vi "MIPI_RFEE_Create Patterns and save to HWS file.vi"(1 "SetID Pin State":u8(ring) items=["0", "1", "Z"], 2 "Mode":enum16{"Write", "Read"}(ring), 5 "file path":path=path "C:/Users/user/Documents/AD2240/Waveforms/RFFE6", 12 "Save .HWS?":bool, 13 "Filename":string) -> ()   [LabVIEW 2013]
doc: "This VI demonstaits how to write to and read back data from a MIPI device. To run this VI:\n1) Change Resource name to the name of your HSDIO card\n2) The MIPI clock will run at <Sample Clock Rate>/<Oversample Factor>. This is 26 MHz (full rate). If your device should be run at a slower rate, decrease the sample clock rate and (or) increase the oversample rate.\n3. At 104MHz, the RTD value should be ~5 for a 1.5 meter cable. If you are running at a different clock rate or using a different length cable, adjust the RTD Compensation value so the MIPI data is stable at the falling edge of the clock. If you need futher timing adjustment, consider setting the data position to \"Delay from Sample Clock Rising Edge\" and configuring this delay."
uses:
  MIPI_RFFE/Ctrls/Configuration.ctl
  MIPI_RFFE/Ctrls/ClockDataChannels.ctl
  MIPI_RFFE/Ctrls/RegReadWrite.ctl
  MIPI_RFFE/Ctrls/ExtendedRegReadWrite.ctl
  <vilib>/Waveform/DWDTOps.llb/Digital Pattern Generator (Single Value).vi
  <vilib>/Waveform/DWDTOps.llb/DWDT Append Digital Signals.vi
  <vilib>/Waveform/DWDTOps.llb/DWDT Append Digital Samples.vi
panel:
  in  "Write Data":T1 {"Register" format="%.0x"; "Slave Address" max=15 format="%.0x"}
  out "Digital Waveform Graph":digitalwaveform(graph)={"t0"=timestamp(3585852840.1106524 s since 1904-01-01), "dt"=5e-07, "Y"={"transitions"=[], "data"=[[1, 0, 1, 0], [1, 0, 1, 0], [1, 0, 1, 0], [1, 0, 1, 0], [1, 0, 1, 0], [1, 0, 1, 0], [1, 0, 1, 0], [1, 0, 1, 0], [0, 0, 0, 0], [0, 0, 0, 0], [0, 0, 0, 0], [0, 0, 0, 0], [0, 0, 0, 0], [0, 0, 0, 0], [0, 0, 0, 0], [0, 0, 0, 0], [0, 1, 0, 1], [0, 1, 0, 1], [0, 1, 0, 1], [0, 1, 0, 1], [0, 0, 0, 0], [0, 0, 0, 0], [0, 0, 0, 0], [0, 0, 0, 0], [1, 1, 1, 1], [1, 1, 1, 1], [1, 1, 1, 1], [1, 1, 1, 1], [1, 0, 1, 0], [1, 0, 1, 0], [1, 0, 1, 0], [1, 0, 1, 0], [1, 1, 1, 1], [1, 1, 1, 1], [1, 1, 1, 1], [1, 1, 1, 1], [1, 0, 1, 0], [1, 0, 1, 0], [1, 0, 1, 0], [1, 0, 1, 0], [0, 1, 0, 1], [0, 1, 0, 1], [0, 1, 0, 1], [0, 1, 0, 1], [0, 0, 0, 0], [0, 0, 0, 0], [0, 0, 0, 0], [0, 0, 0, 0], [0, 1, 0, 1], [0, 1, 0, 1], [0, 1, 0, 1], [0, 1, 0, 1], [0, 0, 0, 0], [0, 0, 0, 0], [0, 0, 0, 0], [0, 0, 0, 0], [1, 1, 1, 1], [1, 1, 1, 1], [1, 1, 1, 1], [1, 1, 1, 1], [1, 0, 1, 0], [1, 0, 1, 0], [1, 0, 1, 0], [1, 0, 1, 0], [0, 1, 0, 1], [0, 1, 0, 1], [0, 1, 0, 1], [0, 1, 0, 1], [0, 0, 0, 0], [0, 0, 0, 0], [0, 0, 0, 0], [0, 0, 0, 0], [1, 1, 1, 1], [1, 1, 1, 1], [1, 1, 1, 1], [1, 1, 1, 1], [1, 0, 1, 0], [1, 0, 1, 0], [1, 0, 1, 0], [1, 0, 1, 0], [1, 1, 1, 1], [1, 1, 1, 1], [1, 1, 1, 1], [1, 1, 1, 1], [1, 0, 1, 0], [1, 0, 1, 0], [1, 0, 1, 0], [1, 0, 1, 0], [1, 1, 1, 1], [1, 1, 1, 1], [1, 1, 1, 1], [1, 1, 1, 1], [1, 0, 1, 0], [1, 0, 1, 0], [1, 0, 1, 0], [1, 0, 1, 0], [0, 1, 0, 1], [0, 1, 0, 1], [0, 1, 0, 1], [0, 1, 0, 1], [0, 0, 0, 0], [0, 0, 0, 0], [0, 0, 0, 0], [0, 0, 0, 0], [0, 1, 0, 1], [0, 1, 0, 1], [0, 1, 0, 1], [0, 1, 0, 1], [0, 0, 0, 0], [0, 0, 0, 0], [0, 0, 0, 0], [0, 0, 0, 0], [1, 1, 1, 1], [1, 1, 1, 1], [1, 1, 1, 1], [1, 1, 1, 1], [1, 0, 1, 0], [1, 0, 1, 0], [1, 0, 1, 0], [1, 0, 1, 0], [1, 1, 1, 1], [1, 1, 1, 1], [1, 1, 1, 1], [1, 1, 1, 1], [1, 0, 1, 0], [1, 0, 1, 0], [1, 0, 1, 0], [1, 0, 1, 0], [0, 1, 0, 1], [0, 1, 0, 1], [0, 1, 0, 1], [0, 1, 0, 1], [0, 0, 0, 0], [0, 0, 0, 0], [0, 0, 0, 0], [0, 0, 0, 0], [0, 1, 0, 1], [0, 1, 0, 1], [0, 1, 0, 1], [0, 1, 0, 1], [0, 0, 0, 0], [0, 0, 0, 0], [0, 0, 0, 0], [0, 0, 0, 0], [0, 1, 0, 1], [0, 1, 0, 1], [0, 1, 0, 1], [0, 1, 0, 1], [0, 0, 0, 0], [0, 0, 0, 0], [0, 0, 0, 0], [0, 0, 0, 0], [0, 1, 0, 1], [0, 1, 0, 1], [0, 1, 0, 1], [0, 1, 0, 1], [0, 0, 0, 0], [0, 0, 0, 0], [0, 0, 0, 0], [0, 0, 0, 0], [0, 1, 0, 1], [0, 1, 0, 1], [0, 1, 0, 1], [0, 1, 0, 1], [0, 0, 0, 0], [0, 0, 0, 0], [0, 0, 0, 0], [0, 0, 0, 0], [0, 1, 0, 1], [0, 1, 0, 1], [0, 1, 0, 1], [0, 1, 0, 1], [0, 0, 0, 0], [0, 0, 0, 0], [0, 0, 0, 0], [0, 0, 0, 0], [0, 1, 0, 1], [0, 1, 0, 1], [0, 1, 0, 1], [0, 1, 0, 1], [0, 0, 0, 0], [0, 0, 0, 0], [0, 0, 0, 0], [0, 0, 0, 0], [0, 1, 0, 1], [0, 1, 0, 1], [0, 1, 0, 1], [0, 1, 0, 1], [0, 0, 0, 0], [0, 0, 0, 0], [0, 0, 0, 0], [0, 0, 0, 0], [0, 1, 0, 1], [0, 1, 0, 1], [0, 1, 0, 1], [0, 1, 0, 1], [0, 0, 0, 0], [0, 0, 0, 0], [0, 0, 0, 0], [0, 0, 0, 0], [1, 0, 1, 0], [1, 0, 1, 0], [1, 0, 1, 0], [1, 0, 1, 0], [1, 0, 1, 0], [1, 0, 1, 0], [1, 0, 1, 0], [1, 0, 1, 0], [0, 0, 0, 0], [0, 0, 0, 0], [0, 0, 0, 0], [0, 0, 0, 0], [0, 0, 0, 0], [0, 0, 0, 0], [0, 0, 0, 0], [0, 0, 0, 0], [0, 1, 0, 1], [0, 1, 0, 1], [0, 1, 0, 1], [0, 1, 0, 1], [0, 0, 0, 0], [0, 0, 0, 0], [0, 0, 0, 0], [0, 0, 0, 0], [1, 1, 1, 1], [1, 1, 1, 1], [1, 1, 1, 1], [1, 1, 1, 1], [1, 0, 1, 0], [1, 0, 1, 0], [1, 0, 1, 0], [1, 0, 1, 0], [1, 1, 1, 1], [1, 1, 1, 1], [1, 1, 1, 1], [1, 1, 1, 1], [1, 0, 1, 0], [1, 0, 1, 0], [1, 0, 1, 0], [1, 0, 1, 0], [0, 1, 0, 1], [0, 1, 0, 1], [0, 1, 0, 1], [0, 1, 0, 1], [0, 0, 0, 0], [0, 0, 0, 0], [0, 0, 0, 0], [0, 0, 0, 0], [0, 1, 0, 1], [0, 1, 0, 1], [0, 1, 0, 1], [0, 1, 0, 1], [0, 0, 0, 0], [0, 0, 0, 0], [0, 0, 0, 0], [0, 0, 0, 0], [1, 1, 1, 1], [1, 1, 1, 1], [1, 1, 1, 1], [1, 1, 1, 1], [1, 0, 1, 0], [1, 0, 1, 0], [1, 0, 1, 0], [1, 0, 1, 0], [1, 1, 1, 1], [1, 1, 1, 1], [1, 1, 1, 1], [1, 1, 1, 1], [1, 0, 1, 0], [1, 0, 1, 0], [1, 0, 1, 0], [1, 0, 1, 0], [1, 1, 1, 1], [1, 1, 1, 1], [1, 1, 1, 1], [1, 1, 1, 1], [1, 0, 1, 0], [1, 0, 1, 0], [1, 0, 1, 0], [1, 0, 1, 0], [1, 1, 1, 1], [1, 1, 1, 1], [1, 1, 1, 1], [1, 1, 1, 1], [1, 0, 1, 0], [1, 0, 1, 0], [1, 0, 1, 0], [1, 0, 1, 0], [1, 1, 1, 1], [1, 1, 1, 1], [1, 1, 1, 1], [1, 1, 1, 1], [1, 0, 1, 0], [1, 0, 1, 0], [1, 0, 1, 0], [1, 0, 1, 0], [0, 1, 0, 1], [0, 1, 0, 1], [0, 1, 0, 1], [0, 1, 0, 1], [0, 0, 0, 0], [0, 0, 0, 0], [0, 0, 0, 0], [0, 0, 0, 0], [0, 1, 0, 1], [0, 1, 0, 1], [0, 1, 0, 1], [0, 1, 0, 1], [0, 0, 0, 0], [0, 0, 0, 0], [0, 0, 0, 0], [0, 0, 0, 0], [0, 1, 0, 1], [0, 1, 0, 1], [0, 1, 0, 1], [0, 1, 0, 1], [0, 0, 0, 0], [0, 0, 0, 0], [0, 0, 0, 0], [0, 0, 0, 0], [0, 1, 0, 1], [0, 1, 0, 1], [0, 1, 0, 1], [0, 1, 0, 1], [0, 0, 0, 0], [0, 0, 0, 0], [0, 0, 0, 0], [0, 0, 0, 0], [1, 1, 5, 1], [1, 1, 5, 1], [1, 1, 5, 1], [1, 1, 5, 1], [1, 0, 4, 0], [1, 0, 5, 0], [1, 0, 5, 0], [1, 0, 5, 0], [0, 1, 5, 1], [0, 1, 5, 1], [0, 1, 5, 1], [0, 1, 5, 1], [0, 0, 3, 0], [0, 0, 5, 0], [0, 0, 5, 0], [0, 0, 5, 0], [0, 1, 5, 1], [0, 1, 5, 1], [0, 1, 5, 1], [0, 1, 5, 1], [0, 0, 3, 0], [0, 0, 5, 0], [0, 0, 5, 0], [0, 0, 5, 0], [0, 1, 5, 1], [0, 1, 5, 1], [0, 1, 5, 1], [0, 1, 5, 1], [0, 0, 3, 0], [0, 0, 5, 0], [0, 0, 5, 0], [0, 0, 5, 0], [0, 1, 5, 1], [0, 1, 5, 1], [0, 1, 5, 1], [0, 1, 5, 1], [0, 0, 3, 0], [0, 0, 5, 0], [0, 0, 5, 0], [0, 0, 5, 0], [0, 1, 5, 1], [0, 1, 5, 1], [0, 1, 5, 1], [0, 1, 5, 1], [0, 0, 3, 0], [0, 0, 5, 0], [0, 0, 5, 0], [0, 0, 5, 0], [0, 1, 5, 1], [0, 1, 5, 1], [0, 1, 5, 1], [0, 1, 5, 1], [0, 0, 3, 0], [0, 0, 5, 0], [0, 0, 5, 0], [0, 0, 5, 0], [0, 1, 5, 1], [0, 1, 5, 1], [0, 1, 5, 1], [0, 1, 5, 1], [0, 0, 3, 0], [0, 0, 5, 0], [0, 0, 5, 0], [0, 0, 5, 0], [0, 1, 5, 1], [0, 1, 5, 1], [0, 1, 5, 1], [0, 1, 5, 1], [0, 0, 3, 0], [0, 0, 5, 0], [0, 0, 5, 0], [0, 0, 5, 0], [0, 1, 0, 1], [0, 1, 0, 1], [0, 1, 0, 1], [0, 1, 0, 1], [0, 0, 0, 0], [0, 0, 0, 0], [0, 0, 0, 0], [0, 0, 0, 0]]}}
  in  "Configuratation":T2={"Samples to Allocate"=10000, "Oversample Factor"=1, "Clock Channel"=enum."0", "Data Channel"=enum."1"} {"Oversample Factor" min=1 max=254; "Samples to Allocate" min=1}
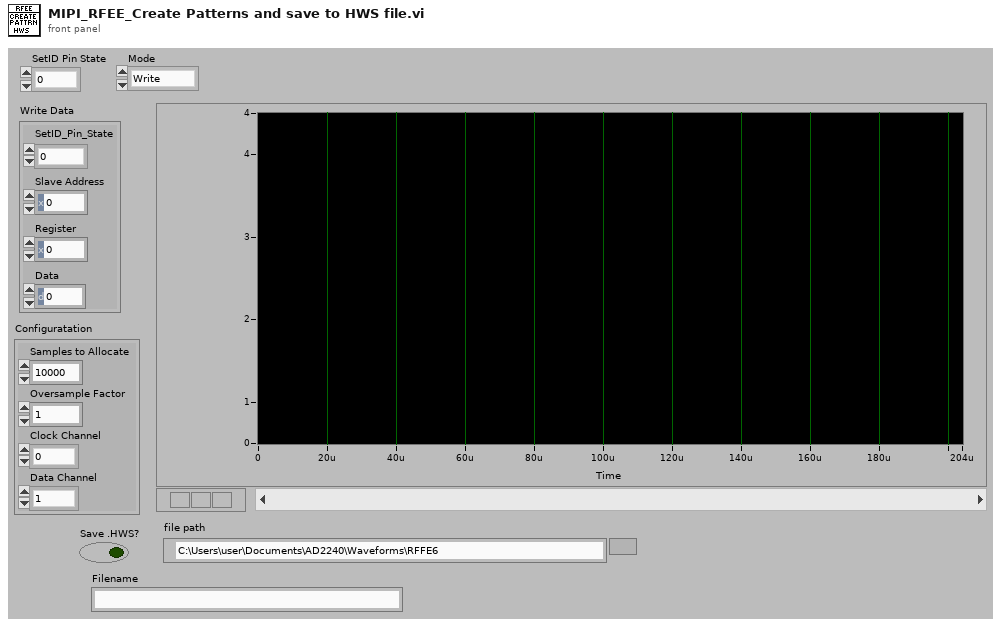
[diagram p1: front panel]
types:
  T1 = typedef "RegReadWrite.ctl" = cluster{"Slave Address":u8, "Register":u8, "Data":u8, "SetID_Pin_State":enum16{"0", "1", "Z"}}
  T2 = typedef "Configuration.ctl" = cluster{"Samples to Allocate":i32, "Oversample Factor":u8, "Clock Channel":T3, "Data Channel":T3}
  T3 = typedef "ClockDataChannels.ctl" = enum16{"0", "1"}
  T4 = typedef "RFFE_Data.ctl" = cluster{"Clock Channel":T3, "Data Channel":T3, "Oversample Factor":u8, "Zero Array":u8[], "One Array":u8[], "Z Array ":u8[], "H Array":u8[], "L Array":u8[], "X Array":u8[], "Toggle (high to low)":u8[]}
  T5 = typedef "ExtendedRegReadWrite.ctl" = cluster{"Slave Address":u8, "Register":u8, "Data":u8[]}
  T6 = typedef "ReadInfo.ctl" = cluster{"Expected Value(s)":u8[], "Compare Locations":u32[]}
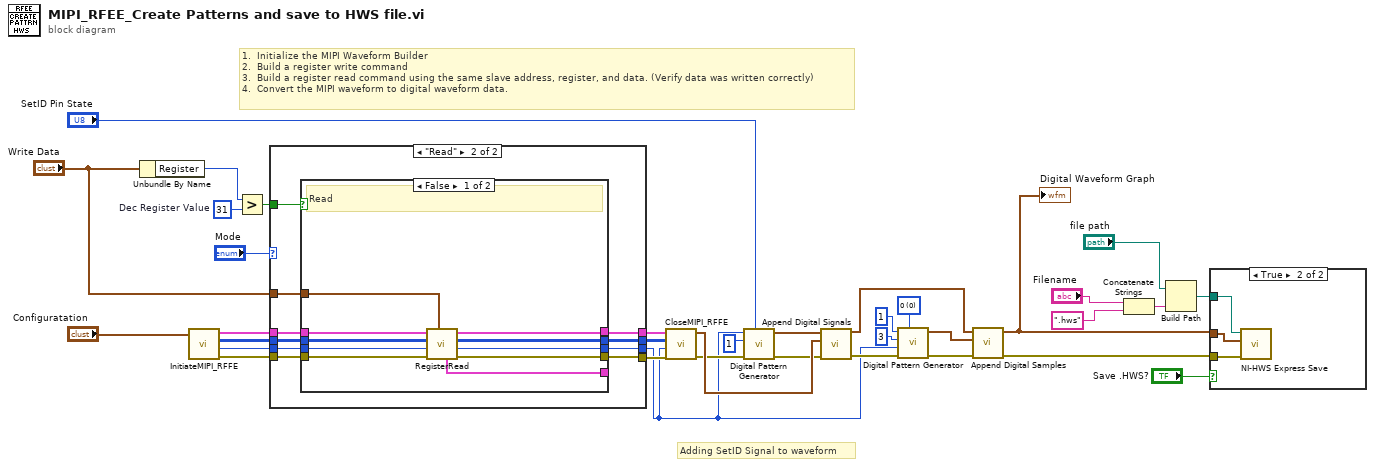
[diagram p0: block diagram]
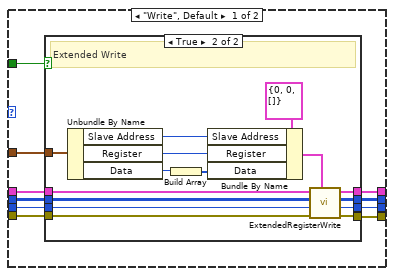
[diagram p2: hidden frame]
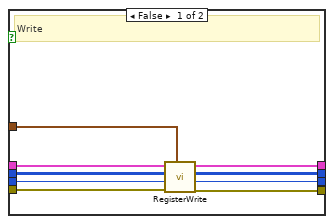
[diagram p3: hidden frame]
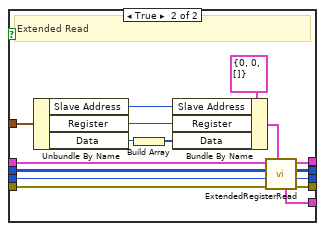
[diagram p4: hidden frame]
diagram:
  w7 = u8 0 items=["0", "1", "Z", "L", "H", "X", "T", "V"] ("value")
  w31 = u8 31  # Dec Register Value
  # "Adding SetID Signal to waveform"
  # "1.  Initialize the MIPI Waveform Builder\n2.  Build a register write command\n3.  Build a register read command using the same slave address, register, and data. (Verify data was written correctly)\n4.  Convert the MIPI waveform to digital waveform data."
  n1 = Unbundle By Name("Write Data") -> ("Register"=w30:u8)
  n2 = call "InitiateMIPI_RFFE.vi"("Configuratation In"="Configuratation") -> ("error out"=w35:errorcluster, "Number of Samples Out"=w34:i32, "Data Array"=w33:u8[][], "RFFE_Data"=w32:T4)  [unwired: 7 in]
  n3 = Greater?(x=w30, y=w31) -> (0:w29:bool)
  n4 = case shown="\"Read\"" "Mode" {
    tunnel: w35 -> [w45 w78]
    tunnel: w34 -> [w44 w75]
    tunnel: w33 -> [w43 w76]
    tunnel: w32 -> [w42 w77]
    tunnel: "Write Data" -> [w41 w70]
    tunnel: w29 -> [w40 w79]
    tunnel: [w39 w71] -> w28
    tunnel: [w38 w72] -> w27
    tunnel: [w37 w74] -> w6
    tunnel: [w36 w73] -> w23
    frame "Write", Default {
      n5 = case shown="True" w40 {
        tunnel: w45 -> [w54 w69]
        tunnel: w44 -> [w53 w66]
        tunnel: w43 -> [w52 w67]
        tunnel: w42 -> [w51 w68]
        tunnel: w41 -> [w46 w64]
        tunnel: [w50 w58] -> w39
        tunnel: [w49 w57] -> w38
        tunnel: [w48 w56] -> w37
        tunnel: [w47 w55] -> w36
        frame False {
          # "Write"
          n6 = call "RegisterWrite.vi"("Write Data"=w46, "error in (no error)"=w54, "Number of Samples In"=w53, "Data Array"=w52, "RFFE_Data"=w51) -> ("error out"=w47:errorcluster, "Number of Samples Out"=w48:i32, "Data Array Out"=w49:u8[][], "Configuratation Out"=w50:T4)  [unwired: 3 in]
        }
        frame True {
          # "Extended Write"
          n7 = Unbundle By Name(w64) -> ("Slave Address"=w63:u8, "Register"=w62:u8, "Data"=w61:u8)
          n8 = Build Array(w61) -> (w60:u8[])
          n9 = Bundle By Name(cluster=T5 {"Slave Address"=0, "Register"=0, "Data"=[]} ("Extended Read/Write"), "Slave Address"=w63, "Register"=w62, "Data"=w60) -> (w59:T5)
          n10 = call "ExtendedRegisterWrite.vi"("Extended Read/Write"=w59, "error in (no error)"=w69, "Number of Samples In"=w66, "Data Array"=w67, "RFFE_Data In"=w68) -> ("error out"=w55:errorcluster, "Number of Samples Out"=w56:i32, "Data Array Out"=w57:u8[][], "RFFE_Data Out"=w58:T4)  [unwired: 3 in]
        }
      }
    }
    frame "Read" {
      n11 = case shown="False" w79 {
        tunnel: [w89 w100] -> w71
        tunnel: [w88 w101] -> w72
        tunnel: [w87 w102] -> w74
        tunnel: [w86 w103] -> w73
        tunnel: [w85 w98] -> _
        tunnel: w78 -> [w84 w90]
        tunnel: w77 -> [w83 w93]
        tunnel: w76 -> [w82 w92]
        tunnel: w75 -> [w81 w91]
        tunnel: w70 -> [w80 w97]
        frame False {
          # "Read"
          n12 = call "RegisterRead.vi"("Register Read/Write"=w80, "error in (no error)"=w84, "Number of Samples In"=w81, "Data Array"=w82, "RFFE_Data In"=w83) -> ("error out"=w86:errorcluster, "Number of Samples Out out"=w87:i32, "Data Array Out"=w88:u8[][], "RFFE_Data Out"=w89:T4, "Compare Bits Out"=w85:T6[])  [unwired: 2 in]
        }
        frame True {
          # "Extended Read"
          n13 = Unbundle By Name(w97) -> ("Slave Address"=w95:u8, "Register"=w96:u8, "Data"=w104:u8)
          n14 = Build Array(w104) -> (w94:u8[])
          n15 = Bundle By Name(cluster=T5 {"Slave Address"=0, "Register"=0, "Data"=[]} ("Extended Read/Write"), "Slave Address"=w95, "Register"=w96, "Data"=w94) -> (w99:T5)
          n16 = call "ExtendedRegisterRead.vi"("Extended Read/Write"=w99, "error in (no error)"=w90, "Number of Samples In"=w91, "Data Array"=w92, "RFFE_Data In"=w93) -> ("error out"=w103:errorcluster, "Number of Samples Out out"=w102:i32, "Data Array Out"=w101:u8[][], "RFFE_Data Out"=w100:T4, "Compare Bits Out"=w98:T6[])  [unwired: 2 in]
        }
      }
    }
  }
  n17 = call "CloseMIPI_RFFE.vi"("error in (no error)"=w23, "Number of Samples"=w6, "Data Array"=w27, "RFFE_Data"=w28) -> ("error out"=w15:errorcluster, "Digital Waveform"=w16:digitalwaveform)  [unwired: 6 in]
  n18 = call-poly <vilib>:"Digital Pattern Generator.vi"("value"="SetID Pin State", "error in (no error)"=w15, "number of signals"=u32 1, "number of samples"=w6) -> ("error out"=w14:errorcluster, "digital waveform"=w17:digitalwaveform)  [unwired: 6 in]
  n19 = call-poly <vilib>:"Append Digital Signals.vi"("error in (no error)"=w14, "digital waveform (low bits)"=w16, "digital waveform (high bits)"=w17) -> ("error out"=w10:errorcluster, "digital waveform out"=w5:digitalwaveform)  [unwired: 7 in]
  n20 = call-poly <vilib>:"Digital Pattern Generator.vi"("value"=w7, "error in (no error)"=w10, "sample rate"=w6, "number of signals"=u32 3, "number of samples"=u32 1) -> ("error out"=w9:errorcluster, "digital waveform"=w4:digitalwaveform)  [unwired: 5 in]
  n21 = call-poly <vilib>:"Append Digital Samples.vi"("error in (no error)"=w9, "digital waveform B"=w4, "digital waveform A"=w5) -> ("error out"=w13:errorcluster, "digital waveform out"=w12:digitalwaveform)  [unwired: 7 in]
  "Digital Waveform Graph" <- w12
  n22 = Concatenate Strings("Filename", ".hws" ("string")) -> (w20:string)
  n23 = Build Path(base path="file path", name or relative path=w20) -> (appended path=w24:path)
  n24 = case shown="True" "Save .HWS?" {
    tunnel: w12 -> [_ w108]
    tunnel: w13 -> [_ w107]
    tunnel: w24 -> [_ w106]
    frame False {
    }
    frame True {
      n25 = call "NI-HWS Express Save"("error in"=w107, "digital waveform"=w108, "file path"=w106) -> ()  [unwired: 8 in, 1 out]
    }
  }
